vi "finalchannelselecthack_focusalign.vi"() -> (1 "devices":u32[](array[numeric]), 2 "Device chans":T1(array[cluster]))   [LabVIEW 2015]
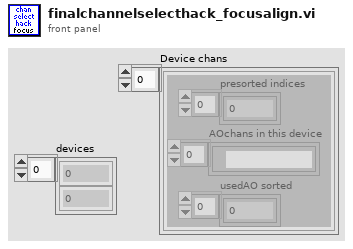
[diagram p1: front panel]
types:
  T1 = cluster{"presorted indices":i32[], "AOchans in this device":tag[], "usedAO sorted":i32[]}[]
  T2 = cluster{"StageS":i32, "StageL":i32, "currmeas data dir":path, "image OD":u16, "contour OD":u16, "point OD":u16, "AOlines":tag[], "AIlines":tag[], "CI lines":tag[], "DO lines":tag[], "AO names":string[], "CI names":string[], "AI names":string[], "DO names":string[], "CIextensions":string[], "AIextensions":string[], "Voltage to Ygalvo":i32, "Voltage to Xgalvo":i32, "Voltage to patch":i32, "640 shutter":i32, "2P shutter":i32, "LT timestamp":u32, "Vp":i32, "Ip":i32, "camera trigger":i32, "master data dir":path, "voltage to Zpos":i32, "Vto2P":i32, "640 AO":i32, "488 AO":i32, "532 AO":i32, "640TTL":u32, "488TTL":u32, "532TTL":u32, "Device 1 sampleclock out":tag, "Device 1 Starttrigger out":tag, "Device 2 sampleclock in":tag, "Device 2 StartTrigger in ":tag, "2PODTTL":u32, "488 shutter":u32, "LCVR red":u32, "LCVR blue":u32}
  T3 = cluster{"presorted indices":i32[], "AOchans in this device":tag[], "usedAO sorted":i32[]}
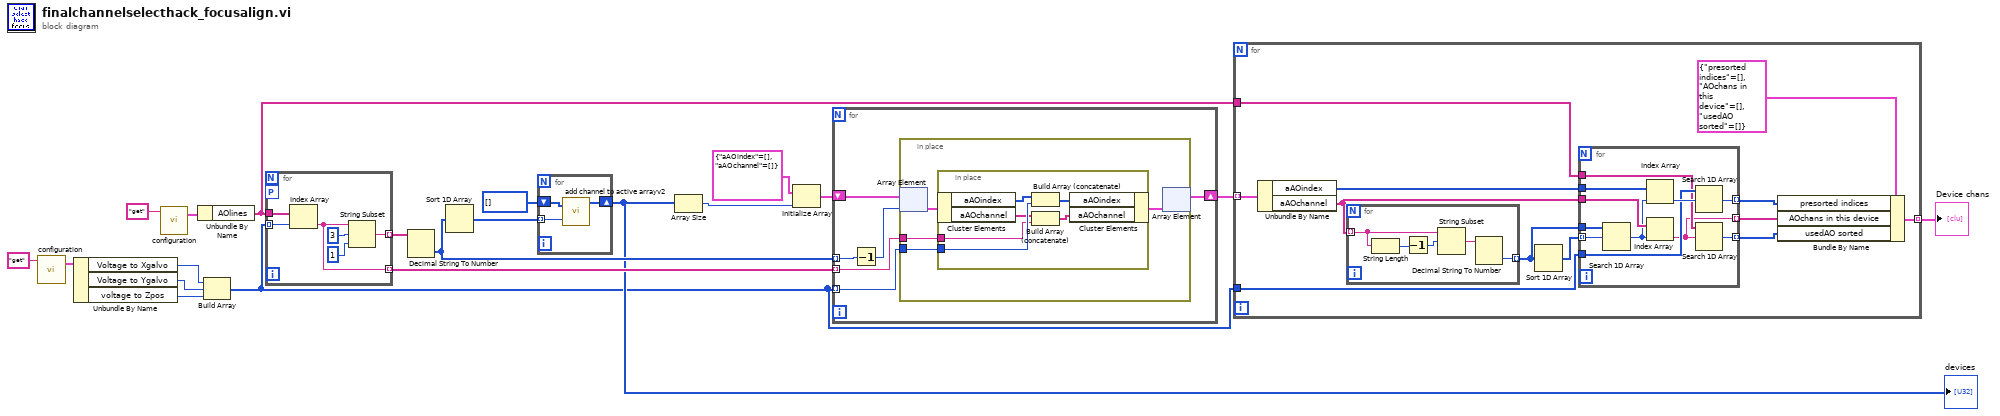
[diagram p0: block diagram]
diagram:
  n1 = call "configuration.vi"("command"="get") -> ("config out"=w6:T2)  [unwired: 2 in, 1 out]
  n2 = Unbundle By Name(w6) -> ("Voltage to Xgalvo"=w4:i32, "Voltage to Ygalvo"=w3:i32, "voltage to Zpos"=w2:i32)
  n3 = call "configuration.vi"("command"="get") -> ("config out"=w19:T2)  [unwired: 2 in, 1 out]
  n4 = Unbundle By Name(w19) -> ("AOlines"=w8:tag[])
  n5 = Build Array(w4, w3, w2) -> (w1:i32[])
  n6 = for {
    tunnel: w1 -> [w25] mode=indexing
    workers-P: _ -> [_]
    tunnel: w8 -> [w26]
    tunnel: [w24] -> w15 mode=indexing
    tunnel: [w21] -> w18 mode=indexing
    n7 = Index Array(array=w26, index=w25) -> (element=w24:tag)
    n8 = String Subset(string=w24, offset (0)=3, length (rest)=1 ("length (rest)")) -> (substring=w21:string)
  }
  n9 = Decimal String To Number(string=w18) -> (number=w14:i32[])  [unwired: 2 in, 1 out]
  n10 = Sort 1D Array(array=w14) -> (sorted array=w16:i32[])
  n11 = for {
    tunnel: w16 -> [w29] mode=indexing
    shift-right: [w27] -> w11
    shift-left: u32[] [] ("line array out") -> [w28]
    n12 = call "add channel to active arrayv2.vi"("line array in"=w28, "line to add"=w29) -> ("line array out"=w27:u32[])  [unwired: 2 out]
  }
  "devices" <- w11
  n13 = Array Size(array=w11) -> (size(s)=w12:i32)
  n14 = Initialize Array(cluster{"aAOindex":u32[], "aAOchannel":tag[]} {"aAOindex"=[], "aAOchannel"=[]} ("Cluster"), w12) -> (w10:cluster{"aAOindex":u32[], "aAOchannel":tag[]}[])
  n15 = for {
    tunnel: w15 -> [w30] mode=indexing
    tunnel: w14 -> [w35] mode=indexing
    tunnel: w1 -> [w31] mode=indexing
    shift-right: [w32] -> w9
    shift-left: w10 -> [w33]
    n16 = Decrement(x=w35) -> (x-1=w34:i32)
    n17 = in-place {
      in-place-border: w31 -> [w37]
      in-place-border: w30 -> [w36]
      n18 = in-place-array #1(w33, w34) -> (w39:cluster{"aAOindex":u32[], "aAOchannel":tag[]})
      n19 = in-place {
        in-place-border: w37 -> [w45]
        in-place-border: w36 -> [w44]
        n20 = in-place-cluster #2(w39) -> ("aAOindex"=w43:u32[], "aAOchannel"=w40:tag[])
        n21 = Build Array (concatenate)(w43, w45) -> (w42:u32[])
        n22 = Build Array (concatenate)(w40, w44) -> (w41:tag[])
        n23 = in-place-cluster #2("aAOindex"=w42, "aAOchannel"=w41) -> (w38:cluster{"aAOindex":u32[], "aAOchannel":tag[]})
      }
      n24 = in-place-array #1(w38) -> (w32:cluster{"aAOindex":u32[], "aAOchannel":tag[]}[])  [unwired: 1 out]
    }
  }
  n25 = for {
    tunnel: w9 -> [w57] mode=indexing
    tunnel: [w52] -> w7 mode=indexing
    tunnel: w1 -> [w50]
    tunnel: w8 -> [w47]
    n26 = Unbundle By Name(w57) -> ("aAOindex"=w51:u32[], "aAOchannel"=w54:tag[])
    n27 = for {
      tunnel: w54 -> [w69] mode=indexing
      tunnel: [w70] -> w55 mode=indexing
      n28 = String Length(string=w69) -> (length=w73:i32)
      n29 = Decrement(x=w73) -> (x-1=w72:i32)
      n30 = String Subset(string=w69, offset (0)=w72) -> (substring=w71:string)  [unwired: 1 in]
      n31 = Decimal String To Number(string=w71) -> (number=w70:i32)  [unwired: 2 in, 1 out]
    }
    n32 = Sort 1D Array(array=w55) -> (sorted array=w56:i32[])
    n33 = for {
      tunnel: w56 -> [w68] mode=indexing
      tunnel: w55 -> [w67]
      tunnel: w54 -> [w66]
      tunnel: [w59] -> w53 mode=indexing
      tunnel: w51 -> [w65]
      tunnel: w50 -> [w63]
      tunnel: [w62] -> w49 mode=indexing
      tunnel: w47 -> [w60]
      tunnel: [w58] -> w46 mode=indexing
      n34 = Search 1D Array(1D array=w67, element=w68) -> (index of element=w61:i32)  [unwired: 1 in]
      n35 = Index Array(array=w65, index=w61) -> (element=w64:u32)
      n36 = Index Array(array=w66, index=w61) -> (element=w59:tag)
      n37 = Search 1D Array(1D array=w63, element=w64) -> (index of element=w62:i32)  [unwired: 1 in]
      n38 = Search 1D Array(1D array=w60, element=w59) -> (index of element=w58:i32)  [unwired: 1 in]
    }
    n39 = Bundle By Name(cluster=T3 {"presorted indices"=[], "AOchans in this device"=[], "usedAO sorted"=[]}, "presorted indices"=w49, "AOchans in this device"=w53, "usedAO sorted"=w46) -> (w52:T3)
  }
  "Device chans" <- w7
